vi "FCE_TS_Action_UpdateChartStyles.vi"(8 "err in":errorcluster) -> (0 "err out":errorcluster)   [LabVIEW 2021]
uses:
  XLP80_General_Libs/WL_Libs_V14.25/WL_Chart_V17.01_mod.llb/WL_Chart_Globals.vi
  XLP80_Globals/Globals_Settings_XLP80.vi
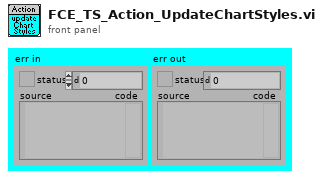
[diagram p1: front panel]
types:
  T1 = cluster{"LineStyle":u8[], "LineWidth":u8[], "LineColor":u32[], "SelectedPlot":i32[], "Scales":u16[], "Enabled":bool[]}
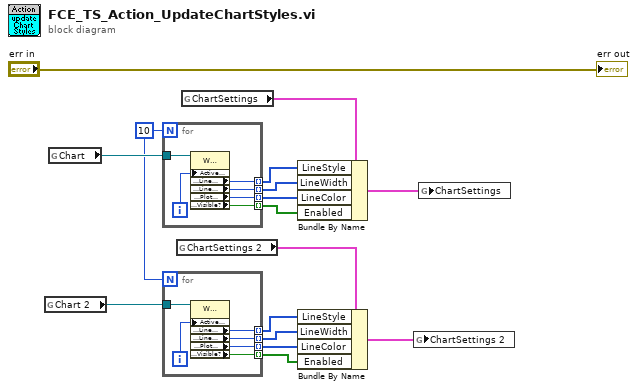
[diagram p0: block diagram]
diagram:
  w7 = 10
  n1 = global read "WL_Chart_Globals.vi" "Chart 2"() -> (w11:refnum<vi>)
  n2 = global read "WL_Chart_Globals.vi" "Chart"() -> (w12:refnum<vi>)
  n3 = for {
    N: w7 -> [_]
    tunnel: w12 -> [w22]
    tunnel: [w20] -> w15 mode=indexing
    tunnel: [w19] -> w14 mode=indexing
    tunnel: [w18] -> w13 mode=indexing
    tunnel: [w17] -> w6 mode=indexing
    i -> [w21]
    n4 = property class="WFChart (strict)"(reference=w22, "Active Plot"=w21) -> ("Plot.Line Style"=w20:u8, "Plot.Line Width"=w19:u8, "Plot.Plot Color"=w18:u32, "Plot.Visible?"=w17:bool)  [unwired: 1 in, 2 out]
  }
  n5 = for {
    N: w7 -> [_]
    tunnel: w11 -> [w28]
    tunnel: [w26] -> w8 mode=indexing
    tunnel: [w25] -> w9 mode=indexing
    tunnel: [w24] -> w10 mode=indexing
    tunnel: [w23] -> w5 mode=indexing
    i -> [w27]
    n6 = property class="WFChart (strict)"(reference=w28, "Active Plot"=w27) -> ("Plot.Line Style"=w26:u8, "Plot.Line Width"=w25:u8, "Plot.Plot Color"=w24:u32, "Plot.Visible?"=w23:bool)  [unwired: 1 in, 2 out]
  }
  n7 = global read "Globals_Settings_XLP80.vi" "ChartSettings 2"() -> (w2:T1)
  n8 = global read "Globals_Settings_XLP80.vi" "ChartSettings"() -> (w4:T1)
  n9 = Bundle By Name(cluster=w4, "LineStyle"=w15, "LineWidth"=w14, "LineColor"=w13, "Enabled"=w6) -> (w3:T1)
  n10 = Bundle By Name(cluster=w2, "LineStyle"=w8, "LineWidth"=w9, "LineColor"=w10, "Enabled"=w5) -> (w1:T1)
  n11 = global write "Globals_Settings_XLP80.vi" "ChartSettings 2"(w1) -> ()
  n12 = global write "Globals_Settings_XLP80.vi" "ChartSettings"(w3) -> ()
  "err out" <- "err in"
